vi "sub vi - send mail with attach v3.vi"(0 "TO:":string, 5 "Attachements":path[](array[path]), 7 "subject":string, 9 "out going server":string, 11 "from":string, 12 "username":string, 13 "password":string) -> (15 "error out":errorcluster)   [LabVIEW 2013]
uses:
  <vilib>/smtpClient/Set Message Text.vi
  <vilib>/smtpClient/LabVIEWSMTPClient.lvlib
panel:
  in  "Array - send address string":string[](array[string])
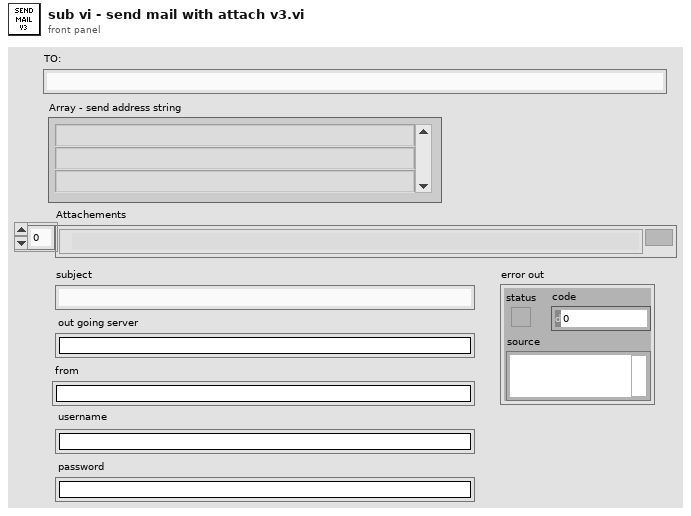
[diagram p1: front panel]
types:
  T1 = typedef "LabVIEWSMTPClient.lvlib/SmtpClientHandle.ctl" = refnum<k1>
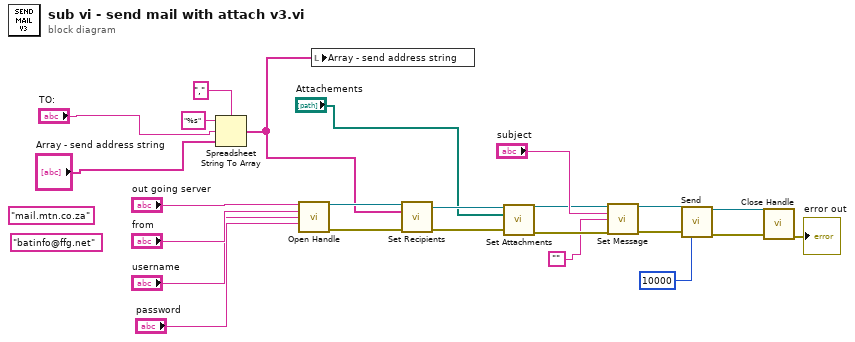
[diagram p0: block diagram]
diagram:
  (unwired) "batinfo@ffg.net"
  (unwired) "mail.mtn.co.za"
  n1 = Spreadsheet String To Array(delimiter (Tab)=",", format string="%s", spreadsheet string="TO:", array type (2D Dbl)="Array - send address string") -> (array=w6:string[])
  n2 = call <vilib>:"Open Handle.vi"("server address"="out going server", "from"="from", "username"="username", "password"="password") -> ("handle out"=w24:T1, "error out"=w23:errorcluster)  [unwired: 10 in]
  n3 = local write "Array - send address string"(w6) -> ()
  n4 = call <vilib>:"Set Recipients.vi"("handle in"=w24, "to"=w6, "error in (no error)"=w23) -> ("handle out"=w22:T1, "error out"=w18:errorcluster)  [unwired: 11 in]
  n5 = call <vilib>:"Set Attachments.vi"("handle in"=w22, "attachments"="Attachements", "error in (no error)"=w18) -> ("handle out"=w20:T1, "error out"=w17:errorcluster)  [unwired: 11 in]
  n6 = call-poly <vilib>:"Set Message.vi"("handle in"=w20, "subject"="subject", "plain text message"="", "error in (no error)"=w17) -> ("handle out"=w19:T1, "error out"=w16:errorcluster)  [unwired: 10 in]
  n7 = call <vilib>:"Send.vi"("handle in"=w19, "error in (no error)"=w16, "timeout in ms (10000)"=10000) -> ("handle out"=w15:T1, "error out"=w14:errorcluster)  [unwired: 10 in, 1 out]
  n8 = call <vilib>:"Close Handle.vi"("handle in"=w15, "error in (no error)"=w14) -> ("error out"=→"error out":errorcluster)  [unwired: 12 in, 1 out]
